vi "Activate Oil Board.vi"(7 "CAN Interface":string, 8 "error in (no error)":errorcluster) -> (0 "error out":errorcluster, 3 "Session Handle out":T1)   [LabVIEW 2015, in "Oil.lvclass"]
uses:
  Oil.lvclass
  Typedefs/Session Handle.ctl
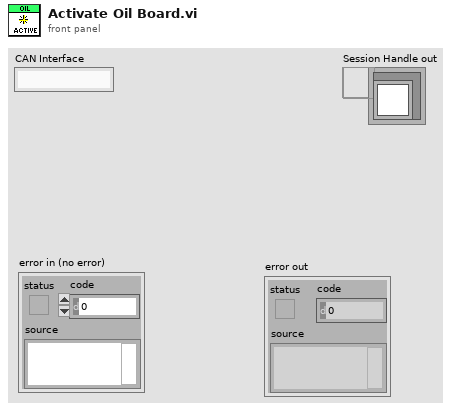
[diagram p1: front panel]
types:
  T1 = typedef "Oil.lvclass/Session Handle.ctl" = refnum<data-value>
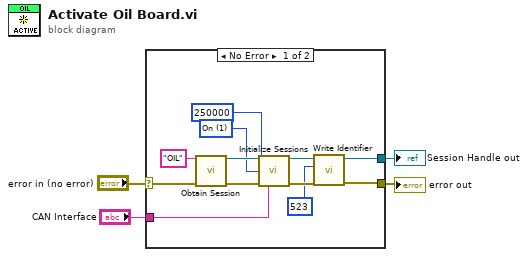
[diagram p0: block diagram]
diagram:
  n1 = case shown="No Error" "error in (no error)" {
    selector: "error in (no error)" -> [w16 w17]
    tunnel: [w8 w17] -> w4
    tunnel: [w6 _] -> w2
    tunnel: "CAN Interface" -> [w5 _]
    frame No Error {
      w11 = u32 1 items=["Off", "On"] ("Termination")
      n2 = call "Obtain Session.vi"("Session  Name ()"="OIL", "error in (no error)"=w16) -> ("Session Handle"=w13:T1, "error out"=w14:errorcluster)  [unwired: 12 in]
      n3 = call "Initialize Sessions.vi"("Session Handle in"=w13, "Baud Rate"=u32 250000, "Termination"=w11, "error in (no error)"=w14, "CAN Interface"=w5) -> ("Session Handle out"=w10:T1, "error out"=w9:errorcluster)  [unwired: 9 in]
      n4 = call "Write Identifier.vi"("error in (no error)"=w9, "identifier"=u32 523, "Session Handle in"=w10) -> ("error out"=w8:errorcluster, "Session Handle out"=w6:T1)  [unwired: 7 in]
    }
    frame Error {
    }
  }
  "error out" <- w4
  "Session Handle out" <- w2
